vi "Asynchronous Call Test.vi"   [LabVIEW 2015]
uses:
  source/library/Scripting.lvlib
  <vilib>/LV-Scripting/LV-Scripting.lvlib
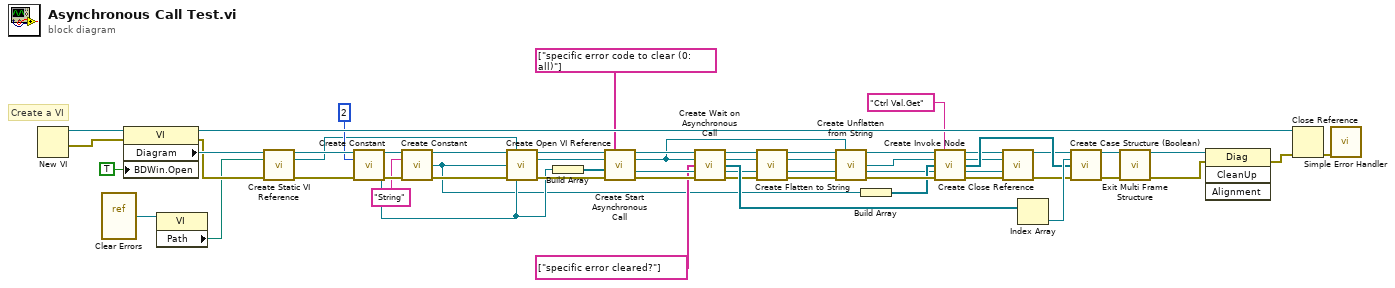
[diagram p0: block diagram]
diagram:
  # "Create a VI"
  n1 = New VI() -> (0:w54:errorcluster, 3:w55:refnum<vi>)  [unwired: 7 in]
  n2 = vi-ref <vilib>:"Clear Errors.vi"() -> (w2:refnum<vi>)
  n3 = property class="VI"(reference=w55, error in=w54, "BDWin.Open"=TRUE ("Block Diagram Window:Open")) -> (reference out=w52:refnum<vi>, error out=w51:errorcluster, "Diagram"=w53:refnum<vi>)
  n4 = property class="VI"(reference=w2) -> ("Path"=w1:path)  [unwired: 1 in, 2 out]
  n5 = call "Create Static VI Reference.vi"("Diagram in"=w53, "VI Path"=w1, "error in (no error)"=w51) -> ("Diagram out"=w46:refnum<vi>, "Terminal"=w27:refnum<vi>, "error out"=w50:errorcluster)  [unwired: 10 in]
  n6 = call <vilib>:"Create Constant.vi"("Diagram in"=w46, "Type"=2, "error in (no error)"=w50) -> ("Diagram out"=w30:refnum<vi>, "Terminal"=w26:refnum<vi>, "error out"=w47:errorcluster)  [unwired: 10 in]
  n7 = call <vilib>:"Create Constant.vi"("Diagram in"=w30, "Type"="String" ("VI Name"), "error in (no error)"=w47) -> ("Diagram out"=w29:refnum<vi>, "Terminal"=w13:refnum<vi>, "error out"=w31:errorcluster)  [unwired: 10 in]
  n8 = call "Create Open VI Reference.vi"("Diagram in"=w29, "type specifier"=w27, "vi path"=w13, "error in (no error)"=w31, "options"=w26) -> ("Diagram out"=w32:refnum<vi>, "vi reference"=w25:refnum<vi>, "error out"=w33:errorcluster)  [unwired: 7 in, 1 out]
  n9 = Build Array(w26) -> (w44:refnum<vi>[])
  n10 = call "Create Start Asynchronous Call.vi"("Diagram in"=w32, "Input Names"=string[] ["specific error code to clear (0: all)"], "reference"=w25, "Inputs"=w44, "error in (no error)"=w33) -> ("Diagram out"=w43:refnum<vi>, "reference out"=w18:refnum<vi>, 10:"error out"=w42:refnum<vi>, 15:"error out"=w49:errorcluster)  [unwired: 7 in]
  n11 = call "Create Wait on Asynchronous Call.vi"("Diagram in"=w43, "reference"=w18, "Output Names"=string[] ["specific error cleared?"], "error in"=w42, "error in (no error)"=w49) -> ("Diagram out"=w23:refnum<vi>, "reference out"=w22:refnum<vi>, "Outputs"=w40:refnum<vi>[], 10:"error out"=w3:refnum<vi>, 15:"error out"=w36:errorcluster)  [unwired: 6 in]
  n12 = call "Create Flatten to String.vi"("Diagram in"=w23, "anything"=w22, "error in"=w3, "error in (no error)"=w36) -> ("Diagram out"=w20:refnum<vi>, "data string"=w19:refnum<vi>, 10:"error out"=w4:refnum<vi>, 15:"error out"=w24:errorcluster)  [unwired: 8 in]
  n13 = call "Create Unflatten from String.vi"("Diagram in"=w20, "type"=w18, "binary string"=w19, "error in"=w4, "error in (no error)"=w24) -> ("Diagram out"=w16:refnum<vi>, "value"=w15:refnum<vi>, 10:"error out"=w5:refnum<vi>, 15:"error out"=w21:errorcluster)  [unwired: 6 in, 1 out]
  n14 = Build Array(w13) -> (w12:refnum<vi>[])
  n15 = call "Create Invoke Node.vi"("Diagram in"=w16, "ID String"="Ctrl Val.Get", "reference"=w15, "Inputs"=w12, "error in"=w5, "error in (no error)"=w21) -> ("Diagram out"=w9:refnum<vi>, "reference out"=w7:refnum<vi>, "Outputs"=w11:refnum<vi>[], 10:"error out"=w6:refnum<vi>, 15:"error out"=w17:errorcluster)  [unwired: 5 in]
  n16 = call "Create Close Reference.vi"("Diagram in"=w9, "application reference"=w7, "error in"=w6, "error in (no error)"=w17) -> ("Diagram out"=w8:refnum<vi>, "error out"=w10:errorcluster)  [unwired: 9 in, 1 out]
  n17 = Index Array(array=w40) -> (element=w37:refnum<vi>)  [unwired: 1 in]
  n18 = call "Create Case Structure (Boolean).vi"("Diagram in"=w8, "Selector"=w37, "Inputs"=w11, "error in (no error)"=w10) -> ("Selected Diagram"=w34:refnum<vi>, "error out"=w35:errorcluster)  [unwired: 8 in, 2 out]
  n19 = call "Exit Multi Frame Structure.vi"("Diagram in"=w34, "error in (no error)"=w35) -> ("Diagram out"=w38:refnum<vi>, "error out"=w39:errorcluster)  [unwired: 11 in, 1 out]
  n20 = invoke class="Diag" method="CleanUp"(reference=w38, error in=w39) -> (error out=w57:errorcluster)  [unwired: 2 in, 3 out]
  n21 = Close Reference(reference=w52, error in (no error)=w57) -> (error out=w56:errorcluster)
  n22 = call <vilib>:"Simple Error Handler.vi"("error in (no error)"=w56) -> ()  [unwired: 4 in, 5 out]
